vi "CTRE_SensoredGearbox_GetPosition.vi"(11 "Sensored Gearbox":T1) -> (2 "Position":dbl, 3 "Sensored Gearbox":T1)   [LabVIEW 2016]
uses:
  <vilib>/Rock Robotics/WPI/ThirdParty/CanMotor/CTRLib-LV-TalonSRX/Framework/SensoredGearbox.ctl
  <vilib>/Rock Robotics/WPI/MotorControl/WPI_MotorControlDeviceRef.ctl
  <vilib>/Rock Robotics/WPI/MotorControl/WPI_MotorControlType.ctl
  <vilib>/Rock Robotics/SystemInterfaces/DIO/FPGA_DIOPWMChannel.ctl
  <vilib>/Rock Robotics/WPI/PWM/WPI_PWMDeadband.ctl
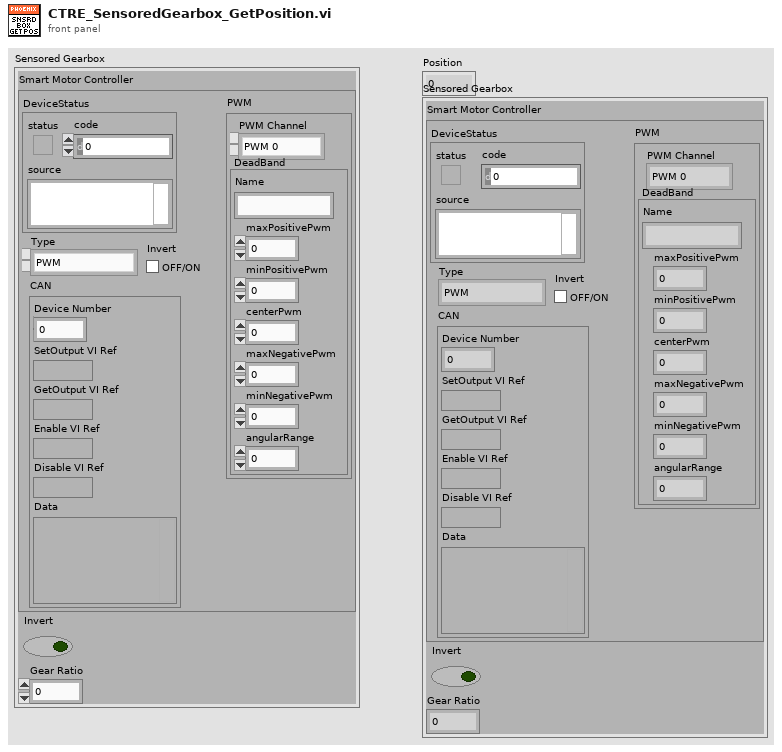
[diagram p1: front panel]
types:
  T1 = typedef "SensoredGearbox.ctl" = cluster{"Smart Motor Controller":T2, "Invert":bool, "Gear Ratio":dbl}
  T2 = typedef "WPI_MotorControlDeviceRef.ctl" = cluster{"DeviceStatus":errorcluster, "Type":T3, "PWM":cluster{"PWM Channel":T4, "DeadBand":T5}, "CAN":cluster{"Device Number":u8, "SetOutput VI Ref":variant, "GetOutput VI Ref":variant, "Enable VI Ref":variant, "Disable VI Ref":variant, "Data":variant}, "Invert":bool}
  T3 = typedef "WPI_MotorControlType.ctl" = enum16{"PWM", "CAN"}
  T4 = typedef "FPGA_DIOPWMChannel.ctl" = enum8{"PWM 0", "PWM 1", "PWM 2", "PWM 3", "PWM 4", "PWM 5", "PWM 6", "PWM 7", "PWM 8", "PWM 9", "PWM MXP 0", "PWM MXP 1", "PWM MXP 2", "PWM MXP 3", "PWM MXP 4", "PWM MXP 5", "PWM MXP 6", "PWM MXP 7", "PWM MXP 8", "PWM MXP 9", "Invalid"}
  T5 = typedef "WPI_PWMDeadband.ctl" = cluster{"Name":string, "maxPositivePwm":i32, "minPositivePwm":i32, "centerPwm":i32, "maxNegativePwm":i32, "minNegativePwm":i32, "angularRange":u16}
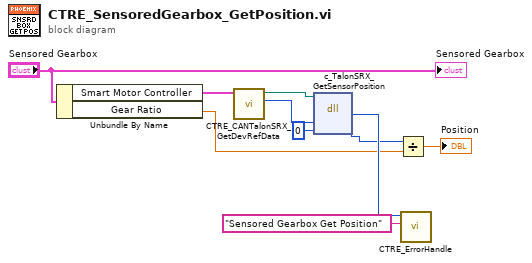
[diagram p0: block diagram]
diagram:
  n1 = Unbundle By Name("Sensored Gearbox") -> ("Smart Motor Controller"=w8:T2, "Gear Ratio"=w1:dbl)
  n2 = call <vilib>:"CTRE_CANTalonSRX_GetDevRefData.vi"("MotorControlDevRef"=w8) -> ("handle"=w6:u64, "Library"=w7:path)  [unwired: 6 in, 3 out]
  n3 = dll-call lib="?" fn="c_TalonSRX_GetSensorPosition"(path in=w7, "m_handle"=w6, "position"=0) -> ("return type"=w4:i32, "position"=w2:i32)  [unwired: 3 in, 2 out]
  n4 = Divide(x=w2, y=w1) -> (x/y=→"Position":dbl)
  n5 = call <vilib>:"CTRE_ErrorHandle.vi"("origin"="Sensored Gearbox Get Position", "code"=w4) -> ()  [unwired: 9 in, 1 out]
  "Sensored Gearbox" <- "Sensored Gearbox"
